vi "Samples per channle (Generation) - Global Variable.vi"() -> ()   [LabVIEW 2018]
panel:
  in  "Samples per channel (Generation)":i32=800
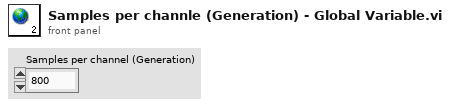
[diagram p1: front panel]
diagram:
